vi "Resize histogram data rolling array.vi"(10 "New max size":i32, 11 "histogram":T1 {"S:" format="%_3f"}) -> (3 "output cluster":T1 {"S:" format="%_3f"})   [LabVIEW 2016]
uses:
  Typedefs/Coincidence single histogram.ctl
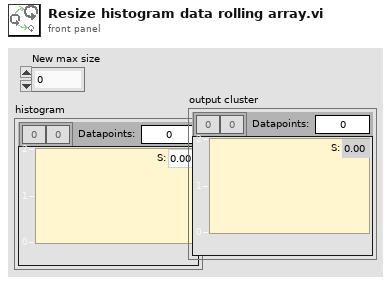
[diagram p1: front panel]
types:
  T1 = typedef "Coincidence single histogram.ctl" = cluster{"Histogram Graph":cluster{"X Values":dbl[], "Histogram: h(x)":i32[]}[], "IDs":i8[], "Datapoints:":i32, "S:":dbl, "Data array":cluster{"Data":i32[], "Max index":i32, "Current index":i32, "Numofpoints":i32}}
  T2 = cluster{"Data":i32[], "Max index":i32, "Current index":i32, "Numofpoints":i32}
  T3 = cluster{"X Values":dbl[], "Histogram: h(x)":i32[]}[]
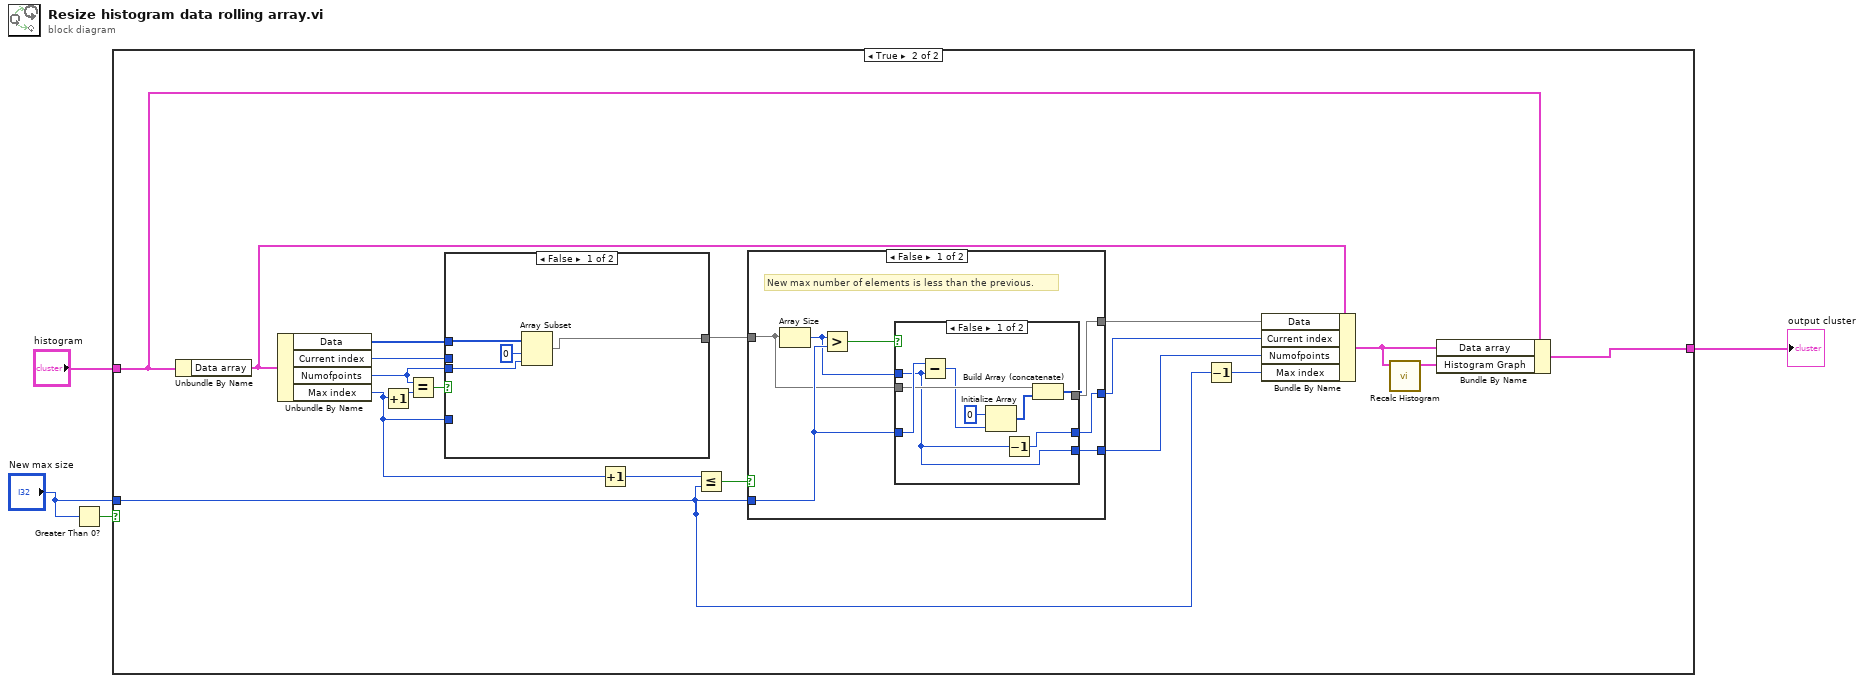
[diagram p0: block diagram]
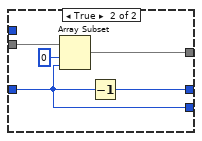
[diagram p3: hidden frame]
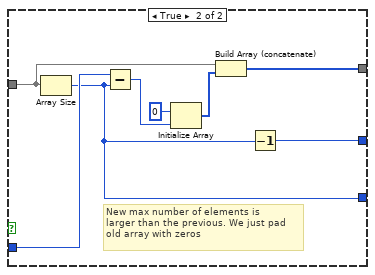
[diagram p4: hidden frame]
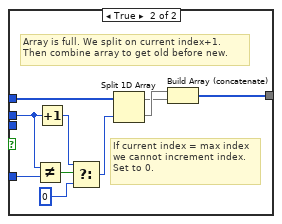
[diagram p5: hidden frame]
diagram:
  n1 = Greater Than 0?(x="New max size") -> (x > 0?=w2:bool)
  n2 = case shown="True" w2 {
    tunnel: "histogram" -> [w5 w15]
    tunnel: [w5 w9] -> w3
    tunnel: "New max size" -> [_ w8]
    frame False {
    }
    frame True {
      n3 = Unbundle By Name(w15) -> ("Data array"=w14:T2)
      n4 = Unbundle By Name(w14) -> ("Data"=w16:i32[], "Current index"=w17:i32, "Numofpoints"=w18:i32, "Max index"=w22:i32)
      n5 = Increment(x=w22) -> (x+1=w19:i32)
      n6 = Equal?(x=w18, y=w19) -> (x = y?=w20:bool)
      n7 = case shown="False" w20 {
        tunnel: w16 -> [w56 w66]
        tunnel: w17 -> [_ w64]
        tunnel: w22 -> [_ w65]
        tunnel: [w53 w57] -> w24
        tunnel: w18 -> [w54 _]
        frame False {
          n8 = Array Subset(array=w56, index=0, length=w54) -> (w53:i32[])
        }
        frame True {
          # "If current index = max index\nwe cannot increment index.\nSet to 0."
          # "Array is full. We split on current index+1.\nThen combine array to get old before new."
          n9 = Not Equal?(x=w64, y=w65) -> (x != y?=w63:bool)
          n10 = Increment(x=w64) -> (x+1=w62:i32)
          n11 = Select(t=w62, s=w63, f=0) -> (s? t:f=w60:i32)
          n12 = Split 1D Array(array=w66, index=w60) -> (first subarray=w58:i32[], second subarray=w59:i32[])
          n13 = Build Array (concatenate)(w59, w58) -> (w57:i32[])
        }
      }
      n14 = Increment(x=w22) -> (x+1=w23:i32)
      n15 = Less Or Equal?(x=w23, y=w8) -> (x <= y?=w21:bool)
      n16 = case shown="False" w21 {
        tunnel: w8 -> [w30 w52]
        tunnel: w24 -> [w27 w48]
        tunnel: [w29 w47] -> w13
        tunnel: [w26 w46] -> w12
        tunnel: [w25 w45] -> w11
        frame False {
          # "New max number of elements is less than the previous."
          n17 = Array Size(array=w27) -> (size(s)=w28:i32)
          n18 = Greater?(x=w28, y=w30) -> (0:w31:bool)
          n19 = case shown="False" w31 {
            tunnel: w27 -> [w35 w44]
            tunnel: w30 -> [w37 w40]
            tunnel: [w36 w42] -> w29
            tunnel: w28 -> [w32 _]
            tunnel: [w34 w41] -> w26
            tunnel: [w32 w40] -> w25
            frame False {
              n20 = Subtract(x=w37, y=w32) -> (x-y=w33:i32)
              n21 = Initialize Array(0 ("element"), w33) -> (w38:i32[])
              n22 = Decrement(x=w32) -> (x-1=w34:i32)
              n23 = Build Array (concatenate)(w35, w38) -> (w36:i32[])
            }
            frame True {
              n24 = Array Subset(array=w44, index=0, length=w40) -> (w42:i32[])
              n25 = Decrement(x=w40) -> (x-1=w41:i32)
            }
          }
        }
        frame True {
          # "New max number of elements is \nlarger than the previous. We just pad \nold array with zeros"
          n26 = Array Size(array=w48) -> (size(s)=w45:i32)
          n27 = Subtract(x=w52, y=w45) -> (x-y=w51:i32)
          n28 = Initialize Array(0 ("element"), w51) -> (w49:i32[])
          n29 = Build Array (concatenate)(w48, w49) -> (w47:i32[])
          n30 = Decrement(x=w45) -> (x-1=w46:i32)
        }
      }
      n31 = Decrement(x=w8) -> (x-1=w10:i32)
      n32 = Bundle By Name(cluster=w14, "Data"=w13, "Current index"=w12, "Numofpoints"=w11, "Max index"=w10) -> (w7:T2)
      n33 = call "Recalc Histogram.vi"("Rolling array in"=w7) -> ("Hist and fit"=w6:T3)  [unwired: 9 in, 1 out]
      n34 = Bundle By Name(cluster=w15, "Data array"=w7, "Histogram Graph"=w6) -> (w9:T1)
    }
  }
  "output cluster" <- w3
